vi "EVENTS(SubVI).vi"() -> (0 "Events":string)   [LabVIEW 2009]
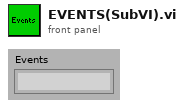
[diagram p1: front panel]
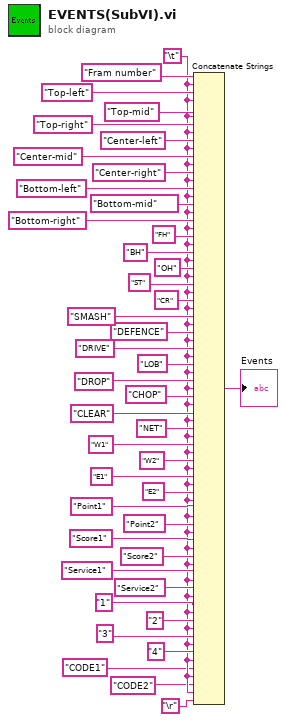
[diagram p0: block diagram]
diagram:
  w4 = "\t"
  n1 = Concatenate Strings("Fram number" ("string"), w4, "Top-left" ("string"), w4, "Top-mid" ("string"), w4, "Top-right" ("string"), w4, "Center-left" ("string"), w4, "Center-mid" ("string"), w4, "Center-right" ("string"), w4, "Bottom-left" ("string"), w4, "Bottom-mid" ("string"), w4, "Bottom-right" ("string"), w4, "FH" ("string"), w4, "BH" ("string"), w4, "OH" ("string"), w4, "ST" ("string"), w4, "CR" ("string"), w4, "SMASH" ("string"), w4, "DEFENCE" ("string"), w4, "DRIVE" ("string"), w4, "LOB" ("string"), w4, "DROP" ("string"), w4, "CHOP" ("string"), w4, "CLEAR" ("string"), w4, "NET" ("string"), w4, "W1" ("string"), w4, "W2" ("string"), w4, "E1" ("string"), w4, "E2" ("string"), w4, "Point1" ("string"), w4, "Point2" ("string"), w4, "Score1" ("string"), w4, "Score2" ("string"), w4, "Service1" ("string"), w4, "Service2" ("string"), w4, "1" ("string"), w4, "2" ("string"), w4, "3" ("string"), w4, "4" ("string"), w4, "CODE1" ("string"), w4, "CODE2" ("string"), w4, "\r") -> (→"Events":string)
